vi "TSM SSC DAQmx Read (Analog 1D Wfm).vi"(0 "DAQ TSM in":T1, 5 "Samples to read":i32=-1, 11 "error in":errorcluster) -> (4 "DAQ TSM Out":T1, 6 "Per-Site Per-Pin Waveforms Out":waveform(dbl)[][](array[waveform]), 15 "error out":errorcluster)   [LabVIEW 2020]
doc: "Reads one or more waveforms from a task that contains one or more analog input channels. The data will be ordered based on the SSC order."
uses:
  Pin Map/TSM DAQmx Multi-Task.ctl
  <vilib>/NI_TestStand_SemiconductorModule/NI_TestStand_Semiconductor_Module.lvlibp/PinMap/PinQueryContext/MultiplePinMultipleSessionQueryContext/MultiplePinMultipleSessionQueryContext.lvclass
  Pin Map/SSC DAQmx.ctl
  4d959a2d-8cc7-4bdb-ba54-34ea8603163a.vi
  Shared SubVIs/Channel List to Pins.vi
  Shared SubVIs/Trim Whitespace [Inlined].vi
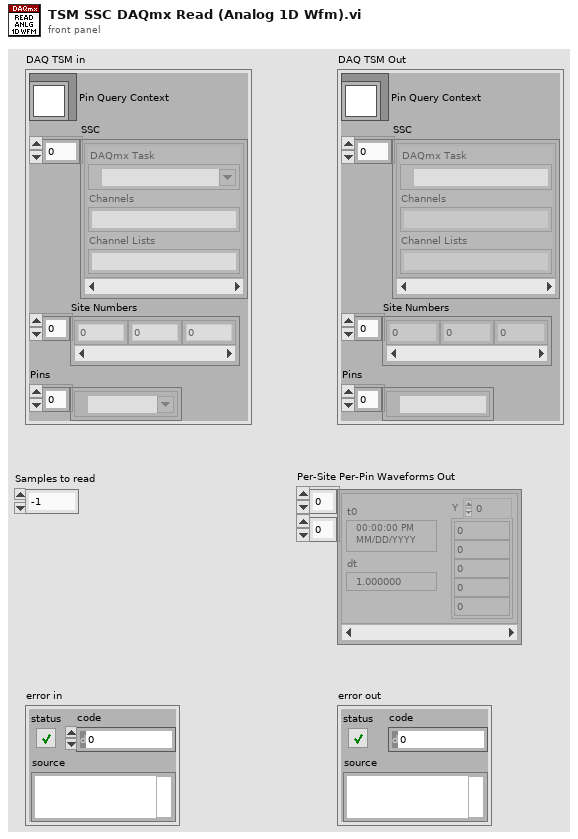
[diagram p1: front panel]
types:
  T1 = typedef "TSM DAQmx Multi-Task.ctl" = cluster{"Pin Query Context":refnum<class "MultiplePinMultipleSessionQueryContext.lvclass">, "SSC":T2[], "Site Numbers":i32[], "Pins":tag[]}
  T2 = typedef "SSC DAQmx.ctl" = cluster{"DAQmx Task ":refnum<k21>, "Channels":string, "Channel Lists":string}
  T3 = typedef "Digital 2D Location Array in a Cluster.ctl" = cluster{"Digital 2D Location Array":T4[]}
  T4 = typedef "Digital 2D Location.ctl" = cluster{"Row":i32, "Col":i32}
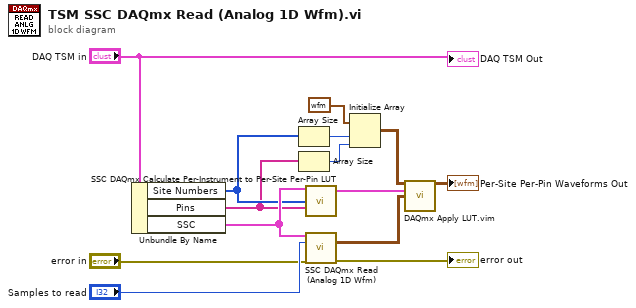
[diagram p0: block diagram]
diagram:
  n1 = Unbundle By Name("DAQ TSM in") -> ("Site Numbers"=w5:i32[], "Pins"=w1:tag[], "SSC"=w6:T2[])
  n2 = Array Size(array=w5) -> (size(s)=w10:i32)
  n3 = Array Size(array=w1) -> (size(s)=w11:i32)
  n4 = call "SSC DAQmx Calculate Per-Instrument to Per-Site Per-Pin LUT.vi"("DAQmx SSC in"=w6, "Sites"=w5, "Pins"=w1) -> ("Per-Task to Per-Site Per-Pin LUT"=w4:T3[])  [unwired: 12 in]
  n5 = call "SSC DAQmx Read (Analog 1D Wfm).vi"("DAQmx SSC in"=w6, "Samples to read"="Samples to read", "error in"="error in") -> ("Per-Task Waveforms out"=w7:waveform(dbl)[][], "error out"=→"error out":errorcluster)  [unwired: 10 in, 1 out]
  n6 = Initialize Array(waveform(dbl) {"t0"=timestamp(0 s since 1904-01-01), "dt"=1.0, "Y"=[]} ("Waveform"), w10, w11) -> (w12:waveform(dbl)[][])
  n7 = call "DAQmx Apply LUT.vim"("Initialized Array"=w12, "LUT"=w4, "Results to Apply LUT to"=w7) -> ("Array Out"=→"Per-Site Per-Pin Waveforms Out":waveform(dbl)[][])  [unwired: 12 in]
  "DAQ TSM Out" <- "DAQ TSM in"
